vi "Get CAN Frame Type Name.vi"(11 "Numeric":u32) -> (3 "String":string)   [LabVIEW 2025, in "CAN-LIN Raw Bus Capture.lvclass"]
uses:
  CAN-LIN Raw Bus Capture.lvclass
  CAN-LIN Raw Bus Capture.lvclass/CAN-LIN Raw Bus Capture.ctl
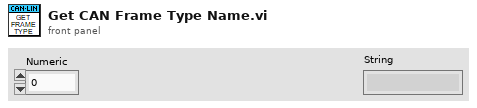
[diagram p1: front panel]
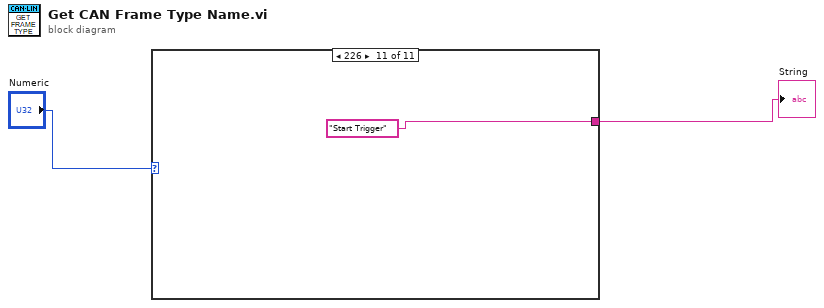
[diagram p0: block diagram]
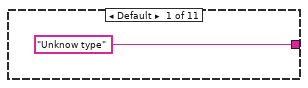
[diagram p2: hidden frame]
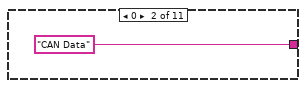
[diagram p3: hidden frame]
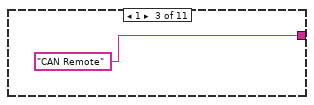
[diagram p4: hidden frame]
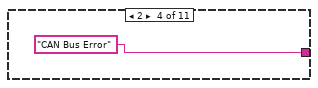
[diagram p5: hidden frame]
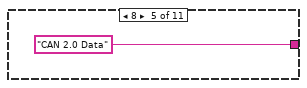
[diagram p6: hidden frame]
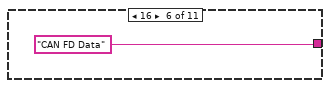
[diagram p7: hidden frame]
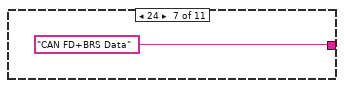
[diagram p8: hidden frame]
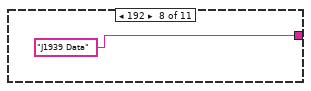
[diagram p9: hidden frame]
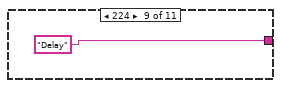
[diagram p10: hidden frame]
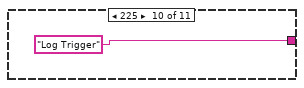
[diagram p11: hidden frame]
diagram:
  n1 = case shown="226" "Numeric" {
    tunnel: ["Unknow type" ("String") "CAN Data" ("String") "CAN Remote" ("String") "CAN Bus Error" ("String") "CAN 2.0 Data" ("String") "CAN FD Data" ("String") "CAN FD+BRS Data" ("String") "J1939 Data" ("String") "Delay" ("String") "Log Trigger" ("String") "Start Trigger" ("String")] -> w1
    frame Default {
    }
    frame 0 {
    }
    frame 1 {
    }
    frame 2 {
    }
    frame 8 {
    }
    frame 16 {
    }
    frame 24 {
    }
    frame 192 {
    }
    frame 224 {
    }
    frame 225 {
    }
    frame 226 {
    }
  }
  "String" <- w1
